vi "InitParameters.vi"(10 "appended path":path) -> (0 "Settings":T1 {"ChkUpdatePeriod" items=["EveryMonth"=2592000, "EveryWeek"=604800, "Everyday"=86400, "EveryHour"=3600, "EveryLaunch"=1, "Never"=0]}, 1 "boolEnableLoadLastDBCbtn":T2(ring), 2 "LastCANpath":path, 3 "LastDBCpath":path)   [LabVIEW 2015]
uses:
  Ctrls/SettingParameters.ctl
  <vilib>/Utility/sysdir.llb/System Directory Type.ctl
  <vilib>/registry/registry.llb/Registry RtKey.ctl
  <vilib>/registry/registry.llb/Registry SAM.ctl
  Ctrls/YesOrNo.ctl
  <vilib>/Utility/config.llb/Write Key (U32).vi
  <vilib>/Utility/config.llb/Read Key (U32).vi
  <vilib>/Utility/config.llb/Write Key (String).vi
  <vilib>/Utility/config.llb/Read Key (String).vi
  <vilib>/Utility/config.llb/Write Key (Double).vi
  <vilib>/Utility/config.llb/Read Key (Double).vi
  <vilib>/Utility/config.llb/Write Key (Boolean).vi
  <vilib>/Utility/config.llb/Read Key (Boolean).vi
  <vilib>/Utility/config.llb/Write Key (Path).vi
  <vilib>/Utility/config.llb/Read Key (Path).vi
  <vilib>/registry/registry.llb/Read Registry Value Simple STR.vi
  GlobalVar.vi
  <vilib>/Utility/config.llb/NI_LVConfig.lvlib
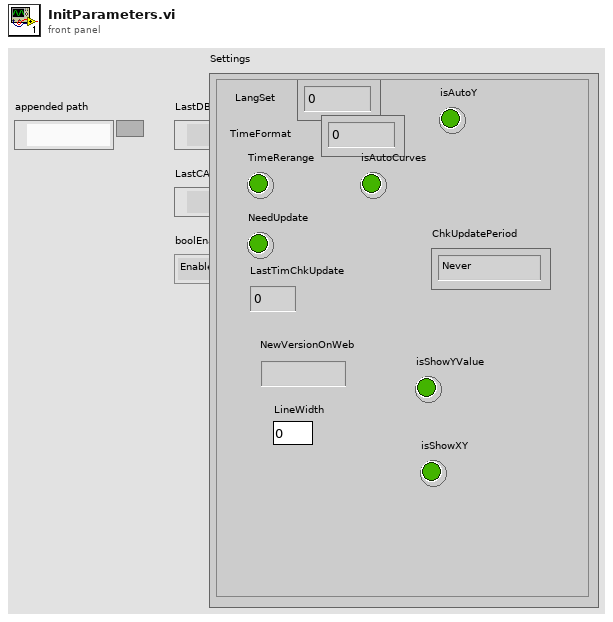
[diagram p1: front panel]
types:
  T1 = typedef "SettingParameters.ctl" = cluster{"LangSet":u32, "TimeFormat":u16, "TimeRerange":bool, "isAutoCurves":bool, "isAutoY":bool, "NeedUpdate":bool, "LastTimChkUpdate":dbl, "NewVersionOnWeb":string, "ChkUpdatePeriod":u32, "LineWidth":u8, "isShowYValue":bool, "isShowXY":bool}
  T2 = enum8{"Enabled", "Disabled", "Disabled and Grayed Out"}
  T3 = typedef "System Directory Type.ctl" = i32
  T4 = typedef "NI_LVConfig.lvlib/Config Data RefNum.ctl" = refnum<k1>
  T5 = typedef "Registry SAM.ctl" = enum32{"KEY_QUERY_VALUE", "KEY_SET_VALUE", "KEY_CREATE_SUB_KEY", "KEY_ENUMERATE_SUB_KEYS", "KEY_NOTIFY", "KEY_CREATE_LINK", "KEY_READ", "KEY_WRITE", "KEY_ALL_ACCESS", "KEY_READ | KEY_WRITE"}
  T6 = typedef "Registry RtKey.ctl" = enum32{"HKEY_CLASSES_ROOT", "HKEY_CURRENT_USER", "HKEY_LOCAL_MACHINE", "HKEY_USERS", "HKEY_PERFORMANCE_DATA", "HKEY_CURRENT_CONFIG", "HKEY_DYN_DATA"}
  T7 = typedef "Registry refnum.ctl" = refnum<k1>
  T8 = typedef "YesOrNo.ctl" = bool
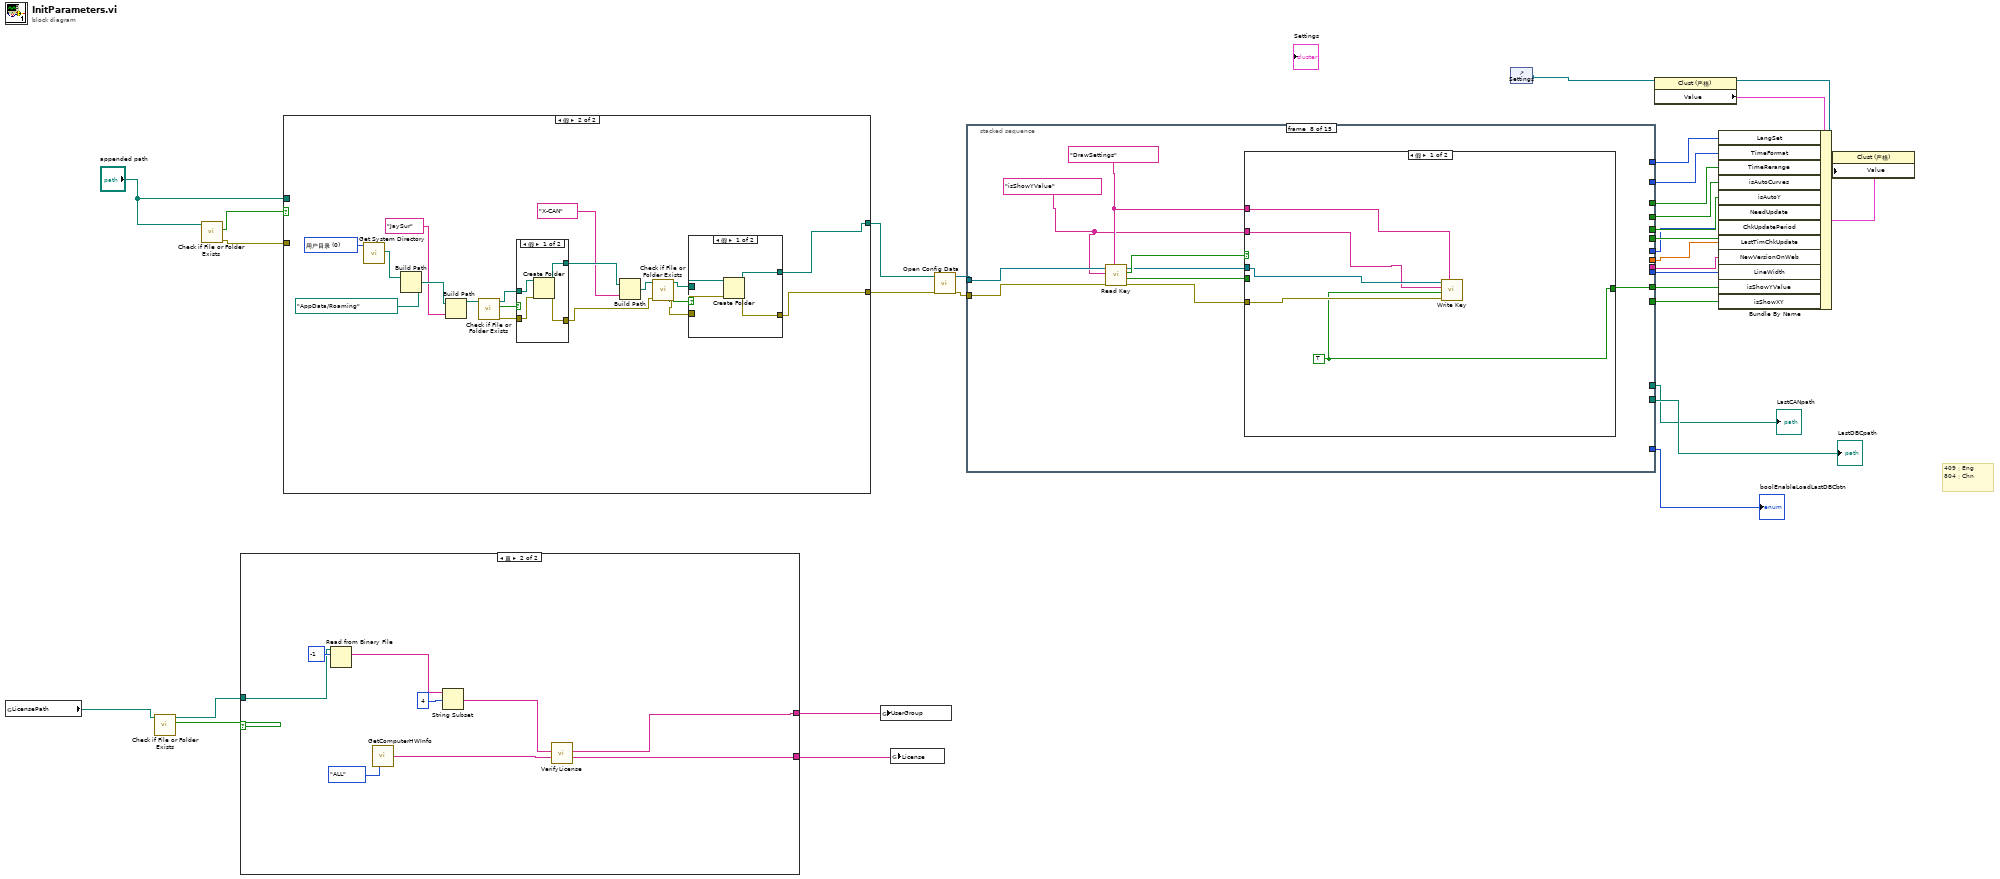
[diagram p0: block diagram]
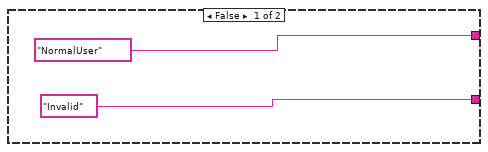
[diagram p2: hidden frame]
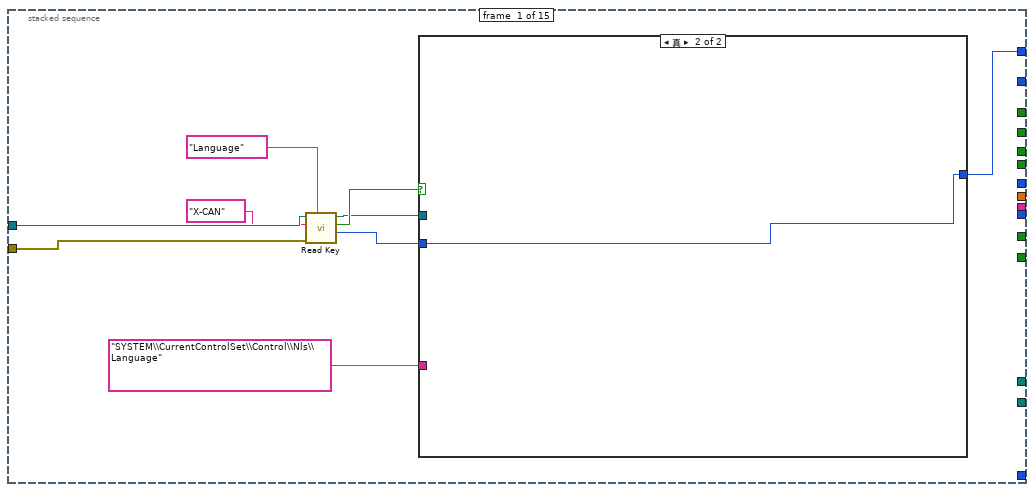
[diagram p3: hidden frame]
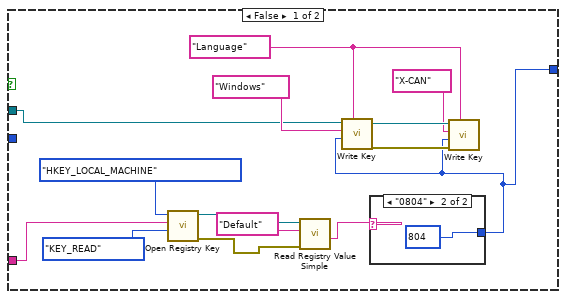
[diagram p4: hidden frame]
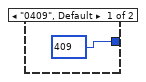
[diagram p5: hidden frame]
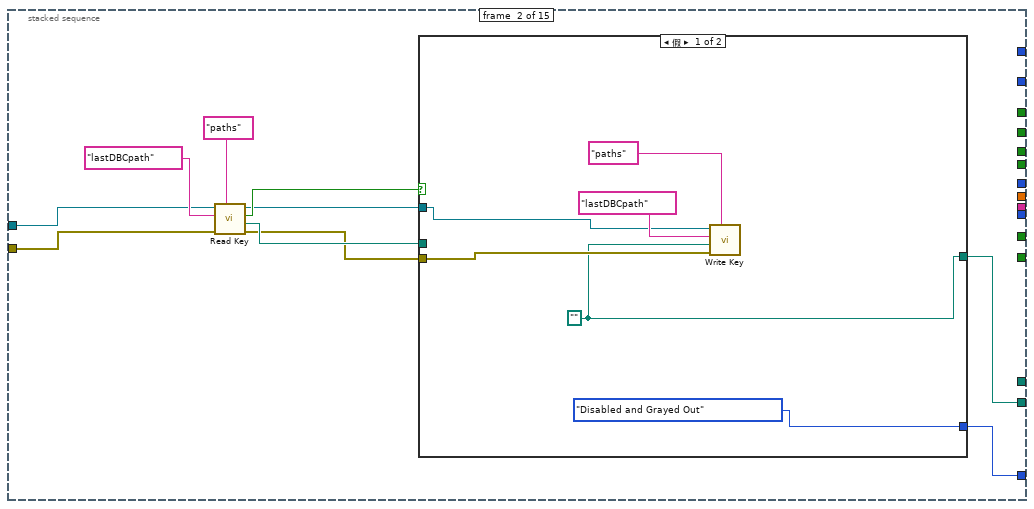
[diagram p6: hidden frame]
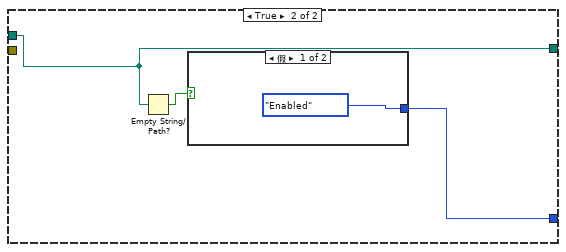
[diagram p7: hidden frame]
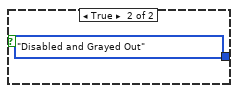
[diagram p8: hidden frame]
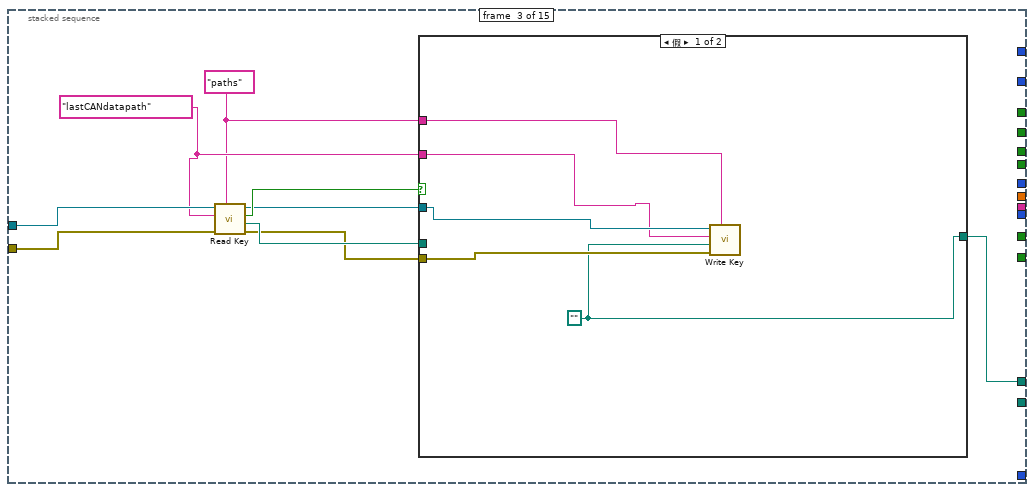
[diagram p9: hidden frame]
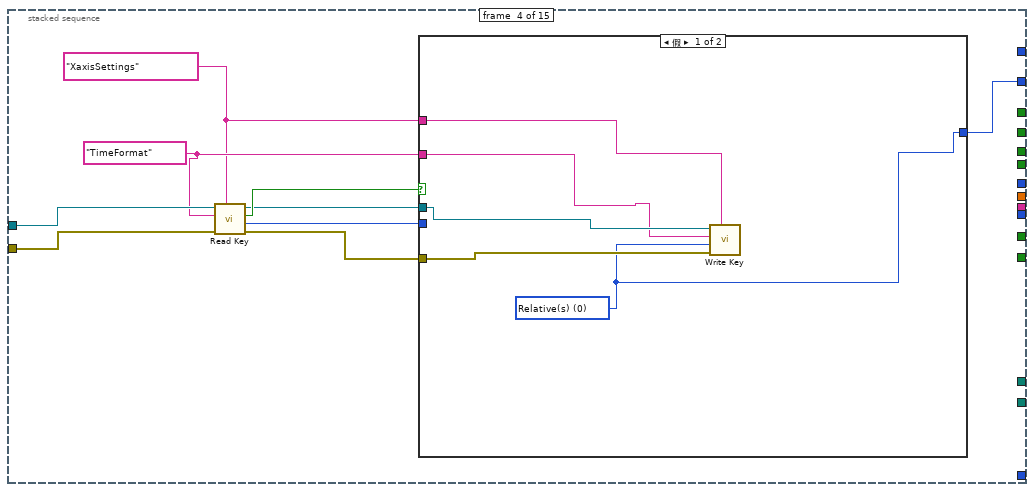
[diagram p11: hidden frame]
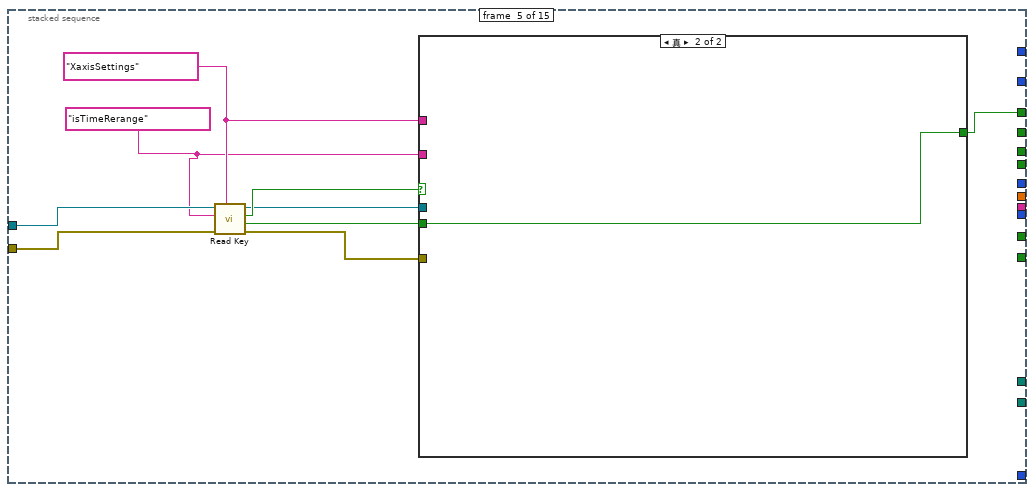
[diagram p13: hidden frame]
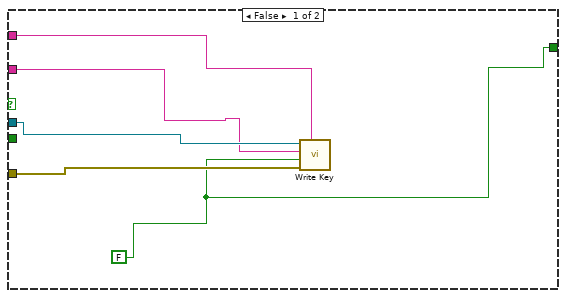
[diagram p14: hidden frame]
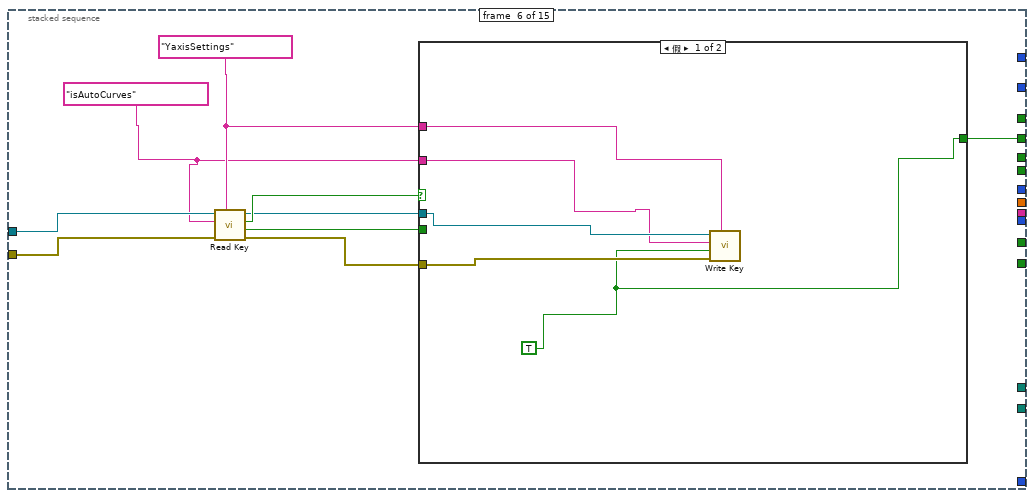
[diagram p15: hidden frame]
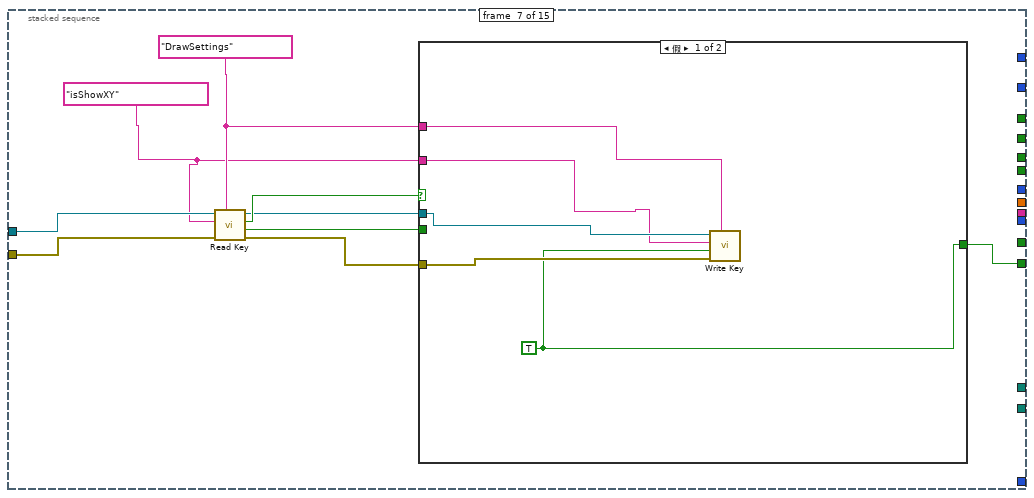
[diagram p17: hidden frame]
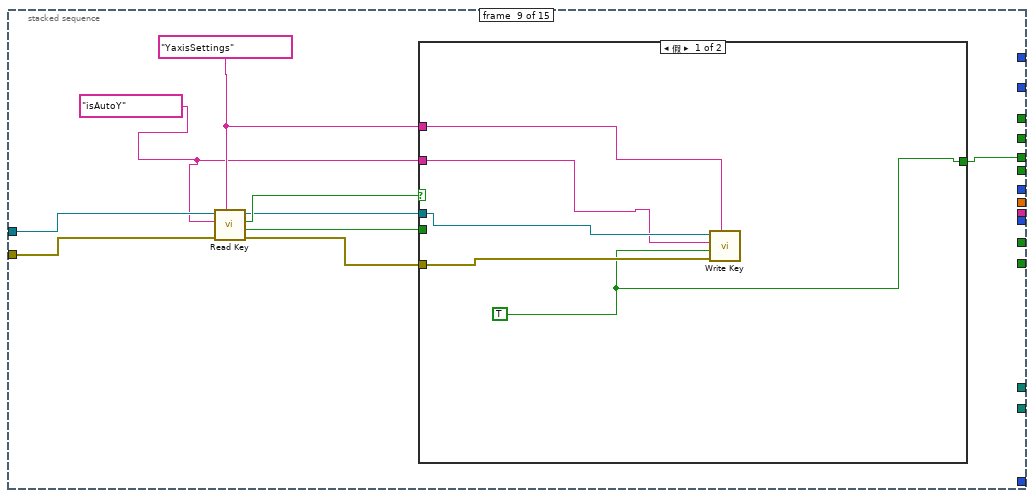
[diagram p20: hidden frame]
diagram:
  # "409：Eng\n804：Chn"
  n1 = global read "GlobalVar.vi" "LicensePath"() -> (w5:path)
  n2 = call <vilib>:"Check if File or Folder Exists.vi"("path"=w5) -> ("file or folder exists?"=w4:bool, "dup path"=w3:path)  [unwired: 8 in, 1 out]
  n3 = call <vilib>:"Check if File or Folder Exists.vi"("path"="appended path") -> ("error out"=w29:errorcluster, "file or folder exists?"=w30:bool)  [unwired: 8 in, 1 out]
  n4 = case shown="真" w4 {
    tunnel: w3 -> [_ w39]
    tunnel: ["NormalUser" w35] -> w2
    tunnel: ["Invalid" w34] -> w1
    frame False {
    }
    frame True {
      n5 = Read from Binary File(10:-1 ("总数(1)"), 11:w39) -> (2:w40:string)  [unwired: 4 in, 3 out]
      n6 = call "GetComputerHWInfo.vi"("获取内容"=enum16{"ALL", "HDD SN", "HDD Type", "MAC Adr"}."ALL") -> ("UID"=w36:string)  [unwired: 13 in, 1 out]
      n7 = String Subset(string=w40, offset (0)=4 ("偏移量(0)")) -> (substring=w37:string)  [unwired: 1 in]
      n8 = call "VerifyLicense.vi"("UID"=w36, "License"=w37) -> ("LicenOut"=w34:string, "user"=w35:string)  [unwired: 8 in]
    }
  }
  n9 = case shown="假" w30 {
    tunnel: "appended path" -> [w44 _]
    tunnel: w29 -> [w43 _]
    tunnel: [w44 w62] -> w25
    tunnel: [w43 w45] -> w24
    frame True {
    }
    frame False {
      w61 = T3 0 items=["用户目录"=0, "用户桌面"=1, "用户文档"=2, "用户应用程序数据"=3, "用户设置"=4, "用户临时目录"=5, "公共文档"=6, "公共应用程序数据"=7, "公共设置"=8, "公共缓存"=13, "系统核心库"=9, "系统安装库"=10, "应用程序文件"=11, "启动盘根目录"=12] ("system directory type")
      n10 = call <vilib>:"Get System Directory.vi"("system directory type"=w61) -> ("system directory"=w59:path)  [unwired: 10 in]
      n11 = Build Path(base path=w59, name or relative path=path "AppData/Roaming" ("default name")) -> (appended path=w58:path)
      n12 = Build Path(base path=w58, name or relative path="JaySur" ("对话框窗口（创建文件夹）")) -> (appended path=w56:path)
      n13 = call <vilib>:"Check if File or Folder Exists.vi"("path"=w56) -> ("error out"=w54:errorcluster, "file or folder exists?"=w55:bool, "dup path"=w53:path)  [unwired: 8 in]
      n14 = case shown="假" w55 {
        tunnel: [w72 w73] -> w52
        tunnel: [w71 w74] -> w49
        tunnel: w54 -> [w70 w74]
        tunnel: w53 -> [w69 w73]
        frame False {
          n15 = Create Folder(path (use dialog)=w69, error in=w70) -> (created path=w72:path, error out=w71:errorcluster)  [unwired: 1 in, 1 out]
        }
        frame True {
        }
      }
      n16 = Build Path(base path=w52, name or relative path="X-CAN" ("对话框窗口（创建文件夹）")) -> (appended path=w50:path)
      n17 = call <vilib>:"Check if File or Folder Exists.vi"("error in (no error)"=w49, "path"=w50) -> ("error out"=w48:errorcluster, "file or folder exists?"=w47:bool, "dup path"=w46:path)  [unwired: 7 in]
      n18 = case shown="假" w47 {
        tunnel: [w66 w67] -> w62
        tunnel: [w65 w68] -> w45
        tunnel: w48 -> [w64 w68]
        tunnel: w46 -> [w63 w67]
        frame False {
          n19 = Create Folder(path (use dialog)=w63, error in=w64) -> (created path=w66:path, error out=w65:errorcluster)  [unwired: 1 in, 1 out]
        }
        frame True {
        }
      }
    }
  }
  n20 = global write "GlobalVar.vi" "UserGroup"(w2) -> ()
  n21 = global write "GlobalVar.vi" "License"(w1) -> ()
  n22 = call <vilib>:"Open Config Data.vi"("error in (no error)"=w24, "configuration file path"=w25) -> ("error out"=w26:errorcluster, "refnum"=w27:T4)  [unwired: 7 in, 1 out]
  n23 = stacked-sequence {
    tunnel: w27 -> [w82 w108 w130 w145 w160 w175 w190 w205 w220 w235 w250 w265 w280 w295 w303]
    tunnel: w26 -> [w79 w107 w129 w144 w159 w174 w189 w204 w219 w234 w249 w264 w279 w294 w302]
    tunnel: [_ w104 _ _ _ _ _ _ _ _ _ _ _ _ _] -> w31
    tunnel: [w75 _ _ _ _ _ _ _ _ _ _ _ _ _ _] -> w20
    tunnel: [_ w103 _ _ _ _ _ _ _ _ _ _ _ _ _] -> w19
    tunnel: [_ _ w124 _ _ _ _ _ _ _ _ _ _ _ _] -> w18
    tunnel: [_ _ _ w137 _ _ _ _ _ _ _ _ _ _ _] -> w17
    tunnel: [_ _ _ _ w152 _ _ _ _ _ _ _ _ _ _] -> w16
    tunnel: [_ _ _ _ _ w169 _ _ _ _ _ _ _ _ _] -> w15
    tunnel: [_ _ _ _ _ _ _ _ w213 _ _ _ _ _ _] -> w14
    tunnel: [_ _ _ _ _ _ _ _ _ w227 _ _ _ _ _] -> w13
    tunnel: [_ _ _ _ _ _ _ _ _ _ w242 _ _ _ _] -> w9
    tunnel: [_ _ _ _ _ _ _ _ _ _ _ w257 _ _ _] -> w11
    tunnel: [_ _ _ _ _ _ _ _ _ _ _ _ w272 _ _] -> w10
    tunnel: [_ _ _ _ _ _ _ _ _ _ _ _ _ w287 _] -> w8
    tunnel: [_ _ _ _ _ _ w182 _ _ _ _ _ _ _ _] -> w7
    tunnel: [_ _ _ _ _ _ _ w197 _ _ _ _ _ _ _] -> w6
    frame #0 {
      n24 = call-poly <vilib>:"Read Key.vi"("section"="Language", "error in (no error)"=w79, "key"="X-CAN", "refnum"=w82) -> ("value"=w78:u32, "found?"=w80:bool, "refnum out"=w77:T4)  [unwired: 4 in, 1 out]
      n25 = case shown="真" w80 {
        tunnel: w78 -> [_ w100]
        tunnel: w77 -> [w86 _]
        tunnel: "SYSTEM\\CurrentControlSet\\Control\\Nls\\Language" ("subkey") -> [w85 _]
        tunnel: [w84 w100] -> w75
        frame False {
          w96 = "Language" ("section")
          n26 = call <vilib>:"Open Registry Key.vi"("security access mask (KEY_READ | KEY_WRITE)"=Registry_SAM."KEY_READ", "subkey"=w85, "root key (HKEY_LOCAL_MACHINE)"=Registry_RtKey."HKEY_LOCAL_MACHINE") -> ("error out"=w88:errorcluster, "refnum out"=w89:T7)  [unwired: 7 in]
          n27 = call-poly <vilib>:"Read Registry Value Simple.vi"("error in (no error)"=w88, "value"="Default", "refnum"=w89) -> ("String/Binary data"=w87:string)  [unwired: 3 in, 3 out]
          n28 = case shown="\"0804\"" w87 {
            tunnel: [u32 409 u32 804] -> w84
            frame "0409", Default {
            }
            frame "0804" {
            }
          }
          n29 = call-poly <vilib>:"Write Key.vi"("section"=w96, "value"=w84, "key"="Windows", "refnum"=w86) -> ("error out"=w97:errorcluster, "refnum out"=w94:T4)  [unwired: 5 in, 1 out]
          n30 = call-poly <vilib>:"Write Key.vi"("section"=w96, "error in (no error)"=w97, "value"=w84, "key"="X-CAN", "refnum"=w94) -> ()  [unwired: 4 in, 3 out]
        }
        frame True {
        }
      }
    }
    frame #1 {
      n31 = call-poly <vilib>:"Read Key.vi"("section"="paths", "error in (no error)"=w107, "key"="lastDBCpath", "refnum"=w108) -> ("error out"=w102:errorcluster, "value"=w105:path, "found?"=w106:bool, "refnum out"=w101:T4)  [unwired: 4 in]
      n32 = case shown="假" w106 {
        tunnel: w105 -> [_ w117]
        tunnel: [T2."Disabled and Grayed Out" ("禁用") w118] -> w104
        tunnel: [w111 w117] -> w103
        tunnel: w102 -> [w113 _]
        tunnel: w101 -> [w112 _]
        frame False {
          w111 = path ""
          n33 = call-poly <vilib>:"Write Key.vi"("section"="paths", "error in (no error)"=w113, "value"=w111, "key"="lastDBCpath", "refnum"=w112) -> ()  [unwired: 4 in, 3 out]
        }
        frame True {
          n34 = Empty String/Path?(string/path=w117) -> (empty?=w119:bool)
          n35 = case shown="假" w119 {
            tunnel: [T2."Enabled" ("禁用") T2."Disabled and Grayed Out" ("禁用")] -> w118
            frame False {
            }
            frame True {
            }
          }
        }
      }
    }
    frame #2 {
      w123 = "lastCANdatapath" ("key")
      w122 = "paths" ("section")
      n36 = call-poly <vilib>:"Read Key.vi"("section"=w122, "error in (no error)"=w129, "key"=w123, "refnum"=w130) -> ("error out"=w126:errorcluster, "value"=w127:path, "found?"=w128:bool, "refnum out"=w125:T4)  [unwired: 4 in]
      n37 = case shown="假" w128 {
        tunnel: w127 -> [_ w136]
        tunnel: [w133 w136] -> w124
        tunnel: w126 -> [w135 _]
        tunnel: w125 -> [w134 _]
        tunnel: w123 -> [w132 _]
        tunnel: w122 -> [w131 _]
        frame False {
          w133 = path ""
          n38 = call-poly <vilib>:"Write Key.vi"("section"=w131, "error in (no error)"=w135, "value"=w133, "key"=w132, "refnum"=w134) -> ()  [unwired: 4 in, 3 out]
        }
        frame True {
        }
      }
    }
    frame #3 {
      w139 = "XaxisSettings" ("section")
      w140 = "TimeFormat" ("key")
      n39 = call-poly <vilib>:"Read Key.vi"("section"=w139, "error in (no error)"=w144, "key"=w140, "refnum"=w145) -> ("error out"=w142:errorcluster, "value"=w138:u32, "found?"=w143:bool, "refnum out"=w141:T4)  [unwired: 4 in]
      n40 = case shown="假" w143 {
        tunnel: w142 -> [w150 _]
        tunnel: w141 -> [w149 _]
        tunnel: w140 -> [w148 _]
        tunnel: w139 -> [w147 _]
        tunnel: w138 -> [_ w151]
        tunnel: [w146 w151] -> w137
        frame False {
          w146 = u16 0 items=["Relative(s)", "Abs(noDate)", "Abs(withDate)"] ("TimeFormat")
          n41 = call-poly <vilib>:"Write Key.vi"("section"=w147, "error in (no error)"=w150, "value"=w146, "key"=w148, "refnum"=w149) -> ()  [unwired: 4 in, 3 out]
        }
        frame True {
        }
      }
    }
    frame #4 {
      w153 = "isTimeRerange" ("key")
      w155 = "XaxisSettings" ("section")
      n42 = call-poly <vilib>:"Read Key.vi"("section"=w155, "error in (no error)"=w159, "key"=w153, "refnum"=w160) -> ("error out"=w157:errorcluster, "value"=w154:bool, "found?"=w158:bool, "refnum out"=w156:T4)  [unwired: 4 in]
      n43 = case shown="真" w158 {
        tunnel: w157 -> [w165 _]
        tunnel: w156 -> [w164 _]
        tunnel: w153 -> [w163 _]
        tunnel: w155 -> [w162 _]
        tunnel: w154 -> [_ w166]
        tunnel: [w161 w166] -> w152
        frame False {
          w161 = T8 FALSE ("isTimeRerange")
          n44 = call-poly <vilib>:"Write Key.vi"("section"=w162, "error in (no error)"=w165, "value"=w161, "key"=w163, "refnum"=w164) -> ()  [unwired: 4 in, 3 out]
        }
        frame True {
        }
      }
    }
    frame #5 {
      w167 = "isAutoCurves" ("key")
      w168 = "YaxisSettings" ("section")
      n45 = call-poly <vilib>:"Read Key.vi"("section"=w168, "error in (no error)"=w174, "key"=w167, "refnum"=w175) -> ("error out"=w172:errorcluster, "value"=w170:bool, "found?"=w173:bool, "refnum out"=w171:T4)  [unwired: 4 in]
      n46 = case shown="假" w173 {
        tunnel: w172 -> [w180 _]
        tunnel: w171 -> [w179 _]
        tunnel: w167 -> [w178 _]
        tunnel: w168 -> [w177 _]
        tunnel: w170 -> [_ w181]
        tunnel: [w176 w181] -> w169
        frame False {
          w176 = T8 TRUE ("isTimeRerange")
          n47 = call-poly <vilib>:"Write Key.vi"("section"=w177, "error in (no error)"=w180, "value"=w176, "key"=w178, "refnum"=w179) -> ()  [unwired: 4 in, 3 out]
        }
        frame True {
        }
      }
    }
    frame #6 {
      w183 = "isShowXY" ("key")
      w184 = "DrawSettings" ("section")
      n48 = call-poly <vilib>:"Read Key.vi"("section"=w184, "error in (no error)"=w189, "key"=w183, "refnum"=w190) -> ("error out"=w187:errorcluster, "value"=w185:bool, "found?"=w188:bool, "refnum out"=w186:T4)  [unwired: 4 in]
      n49 = case shown="假" w188 {
        tunnel: w187 -> [w195 _]
        tunnel: w186 -> [w194 _]
        tunnel: w183 -> [w193 _]
        tunnel: w184 -> [w192 _]
        tunnel: w185 -> [_ w196]
        tunnel: [w191 w196] -> w182
        frame False {
          w191 = T8 TRUE ("isTimeRerange")
          n50 = call-poly <vilib>:"Write Key.vi"("section"=w192, "error in (no error)"=w195, "value"=w191, "key"=w193, "refnum"=w194) -> ()  [unwired: 4 in, 3 out]
        }
        frame True {
        }
      }
    }
    frame #7 {
      w198 = "isShowYValue" ("key")
      w199 = "DrawSettings" ("section")
      n51 = call-poly <vilib>:"Read Key.vi"("section"=w199, "error in (no error)"=w204, "key"=w198, "refnum"=w205) -> ("error out"=w202:errorcluster, "value"=w200:bool, "found?"=w203:bool, "refnum out"=w201:T4)  [unwired: 4 in]
      n52 = case shown="假" w203 {
        tunnel: w202 -> [w210 _]
        tunnel: w201 -> [w209 _]
        tunnel: w198 -> [w208 _]
        tunnel: w199 -> [w207 _]
        tunnel: w200 -> [_ w211]
        tunnel: [w206 w211] -> w197
        frame False {
          w206 = T8 TRUE ("isTimeRerange")
          n53 = call-poly <vilib>:"Write Key.vi"("section"=w207, "error in (no error)"=w210, "value"=w206, "key"=w208, "refnum"=w209) -> ()  [unwired: 4 in, 3 out]
        }
        frame True {
        }
      }
    }
    frame #8 {
      w212 = "isAutoY" ("key")
      w214 = "YaxisSettings" ("section")
      n54 = call-poly <vilib>:"Read Key.vi"("section"=w214, "error in (no error)"=w219, "key"=w212, "refnum"=w220) -> ("error out"=w217:errorcluster, "value"=w215:bool, "found?"=w218:bool, "refnum out"=w216:T4)  [unwired: 4 in]
      n55 = case shown="假" w218 {
        tunnel: w217 -> [w225 _]
        tunnel: w216 -> [w224 _]
        tunnel: w212 -> [w223 _]
        tunnel: w214 -> [w222 _]
        tunnel: w215 -> [_ w226]
        tunnel: [w221 w226] -> w213
        frame False {
          w221 = T8 TRUE ("isTimeRerange")
          n56 = call-poly <vilib>:"Write Key.vi"("section"=w222, "error in (no error)"=w225, "value"=w221, "key"=w223, "refnum"=w224) -> ()  [unwired: 4 in, 3 out]
        }
        frame True {
        }
      }
    }
    frame #9 {
      w228 = "NeedUpdate" ("key")
      w229 = "UpdateSettings" ("section")
      n57 = call-poly <vilib>:"Read Key.vi"("section"=w229, "error in (no error)"=w234, "key"=w228, "refnum"=w235) -> ("error out"=w232:errorcluster, "value"=w230:bool, "found?"=w233:bool, "refnum out"=w231:T4)  [unwired: 4 in]
      n58 = case shown="假" w233 {
        tunnel: w232 -> [w240 _]
        tunnel: w231 -> [w239 _]
        tunnel: w228 -> [w238 _]
        tunnel: w229 -> [w237 _]
        tunnel: w230 -> [_ w241]
        tunnel: [w236 w241] -> w227
        frame False {
          w236 = T8 FALSE ("isTimeRerange")
          n59 = call-poly <vilib>:"Write Key.vi"("section"=w237, "error in (no error)"=w240, "value"=w236, "key"=w238, "refnum"=w239) -> ()  [unwired: 4 in, 3 out]
        }
        frame True {
        }
      }
    }
    frame #10 {
      w243 = "ChkUpdatePeriod" ("key")
      w244 = "UpdateSettings" ("section")
      n60 = call-poly <vilib>:"Read Key.vi"("section"=w244, "error in (no error)"=w249, "key"=w243, "refnum"=w250) -> ("error out"=w247:errorcluster, "value"=w245:u32, "found?"=w248:bool, "refnum out"=w246:T4)  [unwired: 4 in]
      n61 = case shown="假" w248 {
        tunnel: w247 -> [w255 _]
        tunnel: w246 -> [w254 _]
        tunnel: w243 -> [w253 _]
        tunnel: w244 -> [w252 _]
        tunnel: w245 -> [_ w256]
        tunnel: [w251 w256] -> w242
        frame False {
          w251 = u32 1 ("ChkUpdatePeriod")
          # "EveryLaunch"
          n62 = call-poly <vilib>:"Write Key.vi"("section"=w252, "error in (no error)"=w255, "value"=w251, "key"=w253, "refnum"=w254) -> ()  [unwired: 4 in, 3 out]
        }
        frame True {
        }
      }
    }
    frame #11 {
      w258 = "LastTimChkUpdate" ("key")
      w259 = "UpdateSettings" ("section")
      n63 = call-poly <vilib>:"Read Key.vi"("section"=w259, "error in (no error)"=w264, "key"=w258, "refnum"=w265) -> ("error out"=w262:errorcluster, "value"=w260:dbl, "found?"=w263:bool, "refnum out"=w261:T4)  [unwired: 4 in]
      n64 = case shown="假" w263 {
        tunnel: w262 -> [w270 _]
        tunnel: w261 -> [w269 _]
        tunnel: w258 -> [w268 _]
        tunnel: w259 -> [w267 _]
        tunnel: w260 -> [_ w271]
        tunnel: [w266 w271] -> w257
        frame False {
          w266 = 0.0
          n65 = call-poly <vilib>:"Write Key.vi"("section"=w267, "error in (no error)"=w270, "value"=w266, "key"=w268, "refnum"=w269) -> ()  [unwired: 4 in, 3 out]
        }
        frame True {
        }
      }
    }
    frame #12 {
      w273 = "NewVersionOnWeb" ("key")
      w274 = "UpdateSettings" ("section")
      n66 = call-poly <vilib>:"Read Key.vi"("section"=w274, "error in (no error)"=w279, "key"=w273, "refnum"=w280) -> ("error out"=w277:errorcluster, "value"=w275:string, "found?"=w278:bool, "refnum out"=w276:T4)  [unwired: 4 in]
      n67 = case shown="假" w278 {
        tunnel: w277 -> [w285 _]
        tunnel: w276 -> [w284 _]
        tunnel: w273 -> [w283 _]
        tunnel: w274 -> [w282 _]
        tunnel: w275 -> [_ w286]
        tunnel: [w281 w286] -> w272
        frame False {
          w281 = "1.0.0.0"
          n68 = call-poly <vilib>:"Write Key.vi"("section"=w282, "error in (no error)"=w285, "value"=w281, "key"=w283, "refnum"=w284) -> ()  [unwired: 4 in, 3 out]
        }
        frame True {
        }
      }
    }
    frame #13 {
      w288 = "LineWidth" ("key")
      w289 = "LineSettings" ("section")
      n69 = call-poly <vilib>:"Read Key.vi"("section"=w289, "error in (no error)"=w294, "key"=w288, "refnum"=w295) -> ("error out"=w292:errorcluster, "value"=w290:u32, "found?"=w293:bool, "refnum out"=w291:T4)  [unwired: 4 in]
      n70 = case shown="假" w293 {
        tunnel: w292 -> [w300 _]
        tunnel: w291 -> [w299 _]
        tunnel: w288 -> [w298 _]
        tunnel: w289 -> [w297 _]
        tunnel: w290 -> [_ w301]
        tunnel: [w296 w301] -> w287
        frame False {
          w296 = u8 2
          n71 = call-poly <vilib>:"Write Key.vi"("section"=w297, "error in (no error)"=w300, "value"=w296, "key"=w298, "refnum"=w299) -> ()  [unwired: 4 in, 3 out]
        }
        frame True {
        }
      }
    }
    frame #14 {
      n72 = call <vilib>:"Close Config Data.vi"("error in (no error)"=w302, "refnum"=w303) -> ()  [unwired: 8 in, 2 out]
    }
  }
  "boolEnableLoadLastDBCbtn" <- w31
  "LastCANpath" <- w18
  "LastDBCpath" <- w19
  n73 = control-ref of="Settings"() -> (w12:refnum<vi>)
  n74 = property class="Clust (严格)"(reference=w12) -> (reference out=w22:refnum<vi>, "Value"=w21:T1)  [unwired: 1 in, 1 out]
  n75 = Bundle By Name(cluster=w21, "LangSet"=w20, "TimeFormat"=w17, "TimeRerange"=w16, "isAutoCurves"=w15, "isAutoY"=w14, "NeedUpdate"=w13, "ChkUpdatePeriod"=w9, "LastTimChkUpdate"=w11, "NewVersionOnWeb"=w10, "LineWidth"=w8, "isShowYValue"=w6, "isShowXY"=w7) -> (w23:T1)
  n76 = property class="Clust (严格)"(reference=w22, "Value"=w23) -> ()  [unwired: 1 in, 2 out]
